vi "TCP Listener.vi"(8 "error in":errorcluster) -> (0 "error out":errorcluster, 2 "stopped":bool)   [LabVIEW 2020]
uses:
  Device Drivers/shared/stop FGV control.ctl
  Device Driver/shared/FGV_Control.ctl
  Shared/MySQL/Preset Query Enum.ctl
panel:
  out "error out 2":errorcluster
  out "local":bool
  out "remote address":string
  out "Device Name":string
  out "data":string[][](array[string])
  out "element value":string
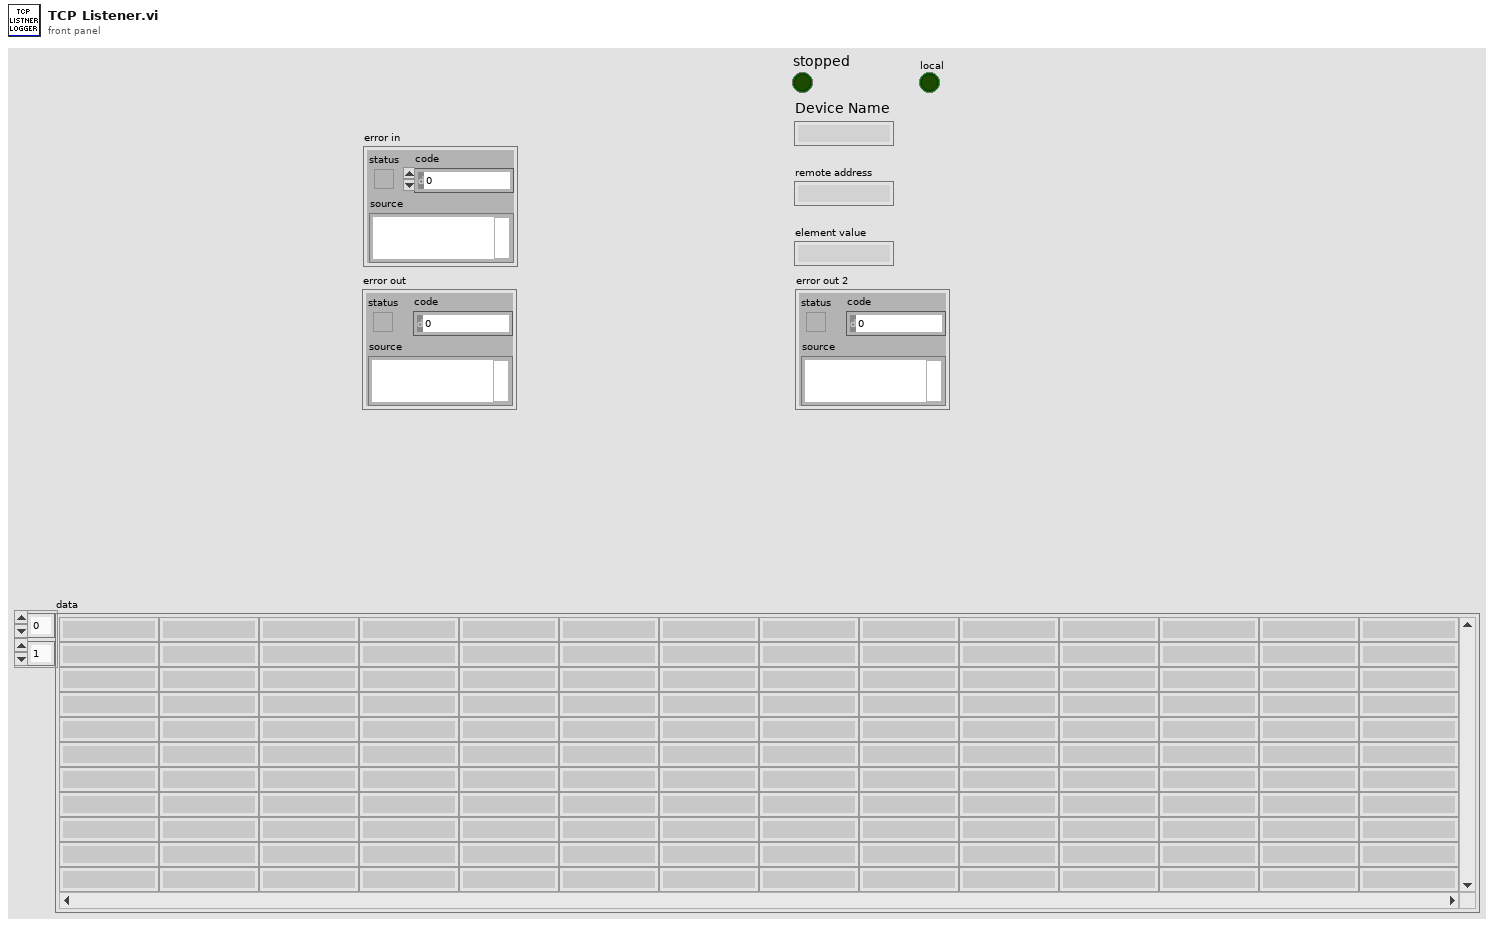
[diagram p1: front panel]
types:
  T1 = typedef "Preset Query Enum.ctl" = enum16{"Get Locations", "Get all IPs and MACs", "Get classes", "Get expt variables to set at scanstart for particular device", "Get expt devices and variables with start values", "Get expt devices and variables (with data to get)", "Get expt devices with data to get", "Get Expt devices and GUIs", "Get all devices basic properties", "Get Virtual Devices Core Info", "Get Expt names", "Get experiment basic properties", "Get experiment alarm variables", "Get MC Ports", "Get device network comm port", "Get devicetype lvclass path", "Get basic device properties", "Get Init Order", "Get all setable variables of a device", "Get device variable aliases", "Get force values of all settable variables", "Get all variables of a devicetype", "Get all variables of a device", "Get plotter details", "Get Saved Scans", "Get Scan Info", "GetGeneralGUIs", "Get expt for plotter", "Get plotter IDs from expt", "Get all devices", "Get all Virtual Devices", "Get all aliases", "Get variable and device info for Virtual Device", "GetItemLocatorIP", "Get IPs for GUIs", "Get DeviceType from Device", "GetLocalPortRange", "GetDevicePresetVariables", "Get Device Configuration", "GetAllPresetNames", "GetAllConfigurationNames", "GetPresetDeviceNames"}
  T2 = typedef "FGV_Control.ctl" = enum16{"add connection", "remove connection", "read variable data", "read connection data", "return all connections", "return all variables", "reset"}
  T3 = typedef "stop FGV control.ctl" = enum16{"Clear", "Write", "Read"}
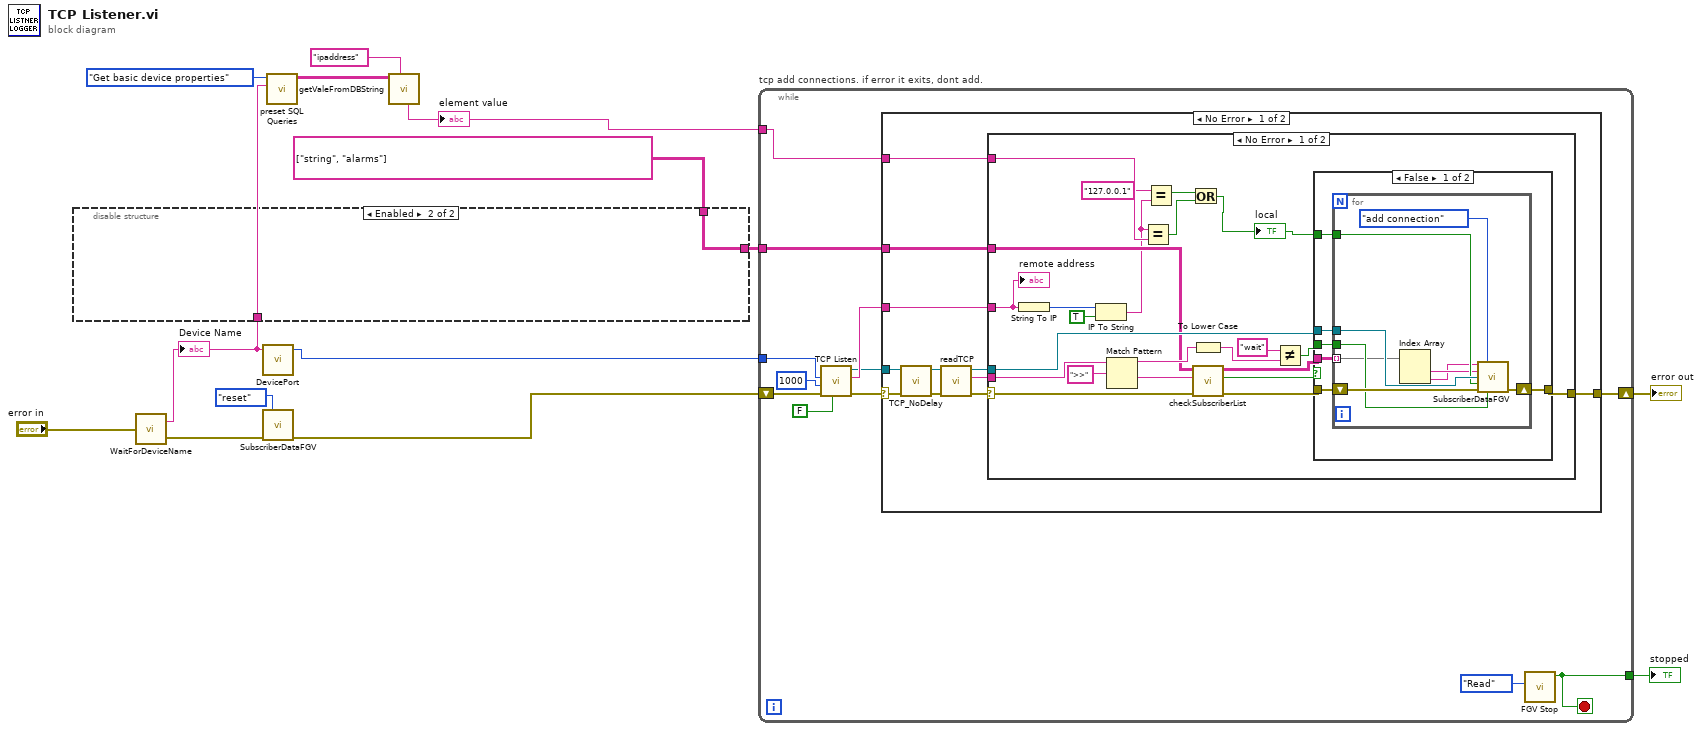
[diagram p0: block diagram]
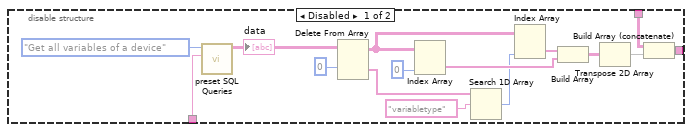
[diagram p2: hidden frame]
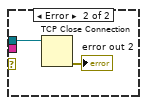
[diagram p4: hidden frame]
diagram:
  n1 = call "WaitForDeviceName.vi"("error in 2"="error in") -> ("Device Name"=w9:string, "error in"=w6:errorcluster)
  "Device Name" <- w9
  n2 = disable-structure shown="Enabled" {
    disable-tunnel: [w29 w30] -> w14
    disable-tunnel: string[][] [["string", "alarms"]] -> [w28 w30]
    disable-tunnel: w9 -> [w26 _]
    frame Disabled {
      n3 = call "preset SQL Queries.vi"("Device/Devicetype name\n/Plotter.id/ScanName#"=w26, "Preset Query"=Preset_Query_Enum."Get all variables of a device") -> ("data"=w17:string[][])  [unwired: 7 in, 2 out]
      "data" <- w17
      n4 = Delete From Array(array=w17, index (row)=0) -> (deleted portion=w19:string[], array with subset deleted=w25:string[][])  [unwired: 2 in]
      n5 = Index Array(array=w25, index (col)=0 ("disabled index (col)")) -> (element=w23:string[])  [unwired: 1 in]
      n6 = Search 1D Array(1D array=w19, element="variabletype") -> (index of element=w21:i32)  [unwired: 1 in]
      n7 = Index Array(array=w25, index (col)=w21) -> (element=w22:string[])  [unwired: 1 in]
      n8 = Build Array(w22, w23) -> (w24:string[][])
      n9 = Transpose 2D Array(2D array=w24) -> (transposed array=w27:string[][])
      n10 = Build Array (concatenate)(w28, w27) -> (w29:string[][])
    }
    frame Enabled {
    }
  }
  n11 = call "DevicePort.vi"("Device Name"=w9) -> ("device port"=w7:u16)  [unwired: 3 in, 1 out]
  n12 = call "SubscriberDataFGV.vi"("command"=FGV_Control."reset", "error in (no error)"=w6) -> ("error out"=w3:errorcluster)  [unwired: 9 in, 4 out]
  n13 = call "preset SQL Queries.vi"("Device/Devicetype name\n/Plotter.id/ScanName#"=w9, "Preset Query"=Preset_Query_Enum."Get basic device properties") -> ("data"=w10:string[][])  [unwired: 7 in, 2 out]
  n14 = call "getValeFromDBString.vi"("element name"="ipaddress" ("element"), "data in"=w10) -> ("element value"=w12:string)  [unwired: 7 in, 2 out]
  "element value" <- w12
  n15 = while "tcp add connections. if error it exits, dont add." {
    tunnel: w7 -> [w42]
    shift-right: [w38] -> w1
    shift-left: w3 -> [w39]
    tunnel: w14 -> [w37]
    tunnel: [w31] -> w4
    tunnel: w12 -> [w35]
    stop <- w31 stop-if-true
    n16 = call <vilib>:"TCP Listen.vi"("resolve remote address (T)"=FALSE, "error in (no error)"=w39, "timeout ms (wait forever: -1)"=1000, "port"=w42) -> ("error out"=w33:errorcluster, "remote address"=w41:string, "connection ID"=w32:refnum<k5>)  [unwired: 3 in, 2 out]
    n17 = case shown="No Error" w33 {
      selector: w33 -> [w45 _]
      tunnel: w41 -> [w49 _]
      tunnel: [w51 _] -> w38
      tunnel: w37 -> [w50 _]
      tunnel: w35 -> [w48 _]
      tunnel: w32 -> [w44 _]
      frame No Error {
        n18 = call "TCP_NoDelay.vi"("error in (no error)"=w45, "connID"=w44) -> ("error out"=w46:errorcluster, "connID 2"=w47:refnum<k5>)  [unwired: 4 in]
        n19 = call "readTCP.vi"("error in (no error)"=w46, "connection ID in"=w47) -> ("error out"=w43:errorcluster, "data out"=w53:string, "connection ID out"=w52:refnum<k5>)  [unwired: 7 in]
        n20 = case shown="No Error" w43 {
          selector: w43 -> [w59 _]
          tunnel: w53 -> [w76 _]
          tunnel: w52 -> [w71 w93]
          tunnel: [w70 _] -> w51
          tunnel: w50 -> [w68 _]
          tunnel: w49 -> [w63 _]
          tunnel: w48 -> [w60 _]
          frame No Error {
            n21 = String To IP(1:w63) -> (0:w62:u32)
            n22 = IP To String(1:TRUE ("dot notation? (F)"), 2:w62) -> (0:w58:string)
            n23 = Match Pattern(string=w76, regular expression=">>") -> (before substring=w72:string, after substring=w67:string)  [unwired: 1 in, 2 out]
            n24 = Equal?(x=w58, y=w60) -> (x = y?=w55:bool)
            n25 = Equal?(x="127.0.0.1", y=w58) -> (x = y?=w56:bool)
            n26 = Or(x=w56, y=w55) -> (x .or. y?=w54:bool)
            "local" <- w54
            n27 = To Lower Case(string=w72) -> (all lower case string=w73:string)
            n28 = call "checkSubscriberList.vi"("error in"=w59, "variable(s)"=w67, "variable type and name"=w68) -> ("error out"=w66:errorcluster, "invalid connection"=w65:bool, "variable and names out"=w64:string[][])  [unwired: 6 in]
            n29 = Not Equal?(x="wait", y=w73) -> (x != y?=w69:bool)
            n30 = case shown="False" w65 {
              tunnel: w71 -> [w82 _]
              tunnel: w54 -> [w81 _]
              tunnel: [w80 _] -> w70
              tunnel: w69 -> [w79 _]
              tunnel: w66 -> [w78 _]
              tunnel: w64 -> [w77 _]
              frame False {
                n31 = for {
                  tunnel: w82 -> [w91]
                  tunnel: w81 -> [w90]
                  shift-right: [w88] -> w80
                  shift-left: w78 -> [w89]
                  tunnel: w79 -> [w87]
                  tunnel: w77 -> [w86] mode=indexing
                  n32 = Index Array(array=w86) -> (element #1=w85:string, element #2=w84:string)  [unwired: 2 in]
                  n33 = call "SubscriberDataFGV.vi"("variable"=w84, "command"=FGV_Control."add connection", "variable type"=w85, "connection ID"=w91, "local"=w90, "error in (no error)"=w89, "spawn"=w87) -> ("error out"=w88:errorcluster)  [unwired: 4 in, 4 out]
                }
              }
              frame True {
              }
            }
            "remote address" <- w63
          }
          frame Error {
            n34 = TCP Close Connection(connection ID=w93) -> (error out=→"error out 2":errorcluster)  [unwired: 2 in, 1 out]
          }
        }
      }
      frame Error {
      }
    }
    n35 = call "FGV Stop.vi"("Function"=stop_FGV_control."Read") -> ("stop out"=w31:bool)  [unwired: 9 in, 1 out]
  }
  "error out" <- w1
  "stopped" <- w4
